vi "IMU Get Acceleration.vi"(8 "error in":errorcluster) -> (0 "error out":errorcluster, 2 "timestamp":i64, 3 "acceleration":cluster{"x":dbl, "y":dbl, "z":dbl}(graph))   [LabVIEW 2026, in "MrcLib.lvlib"]
doc: "Returns the current accelerations of the built-in sensor."
uses:
  MrcLib.lvlib
  Types/MRC 3D Acceleration Values.ctl
panel:
  out "acceleration":T1
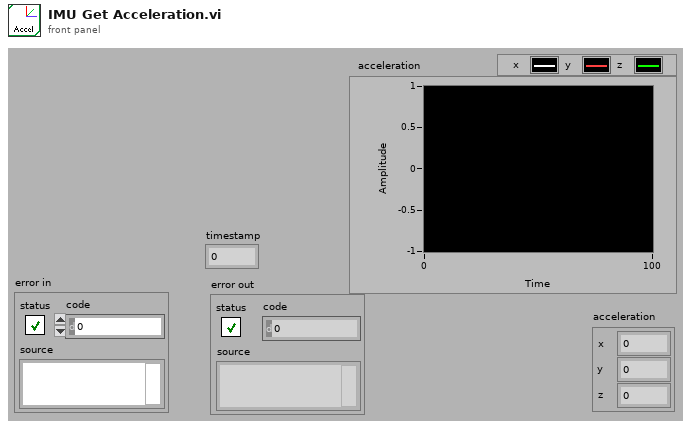
[diagram p1: front panel]
types:
  T1 = typedef "MrcLib.lvlib/MRC 3D Acceleration Values.ctl" = cluster{"x":dbl, "y":dbl, "z":dbl}
  T2 = typedef "MrcLib.lvlib/MRC 3D Acceleration.ctl" = cluster{"timestamp":i64, "x":dbl, "y":dbl, "z":dbl}
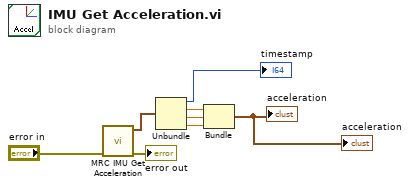
[diagram p0: block diagram]
diagram:
  n1 = call "MRC IMU Get Acceleration.vi"("error in (no error)"="error in") -> ("error out"=→"error out":errorcluster, "acceleration"=w7:T2)  [unwired: 9 in]
  n2 = Unbundle(w7) -> ("timestamp"=→"timestamp":i64, "x"=w6:dbl, "y"=w4:dbl, "z"=w5:dbl)
  n3 = Bundle("x"=w6, "y"=w4, "z"=w5) -> (→"acceleration" →"acceleration":cluster{"x":dbl, "y":dbl, "z":dbl})  [unwired: 1 in]
